vi "CaculateDivergenceAngle .vi"(3 "位置路径":path[](array[path])) -> (0 "纵向发散角":dbl, 1 "横向发散角":dbl)   [LabVIEW 2018]
panel:
  out "Image":T1(plugin-control)
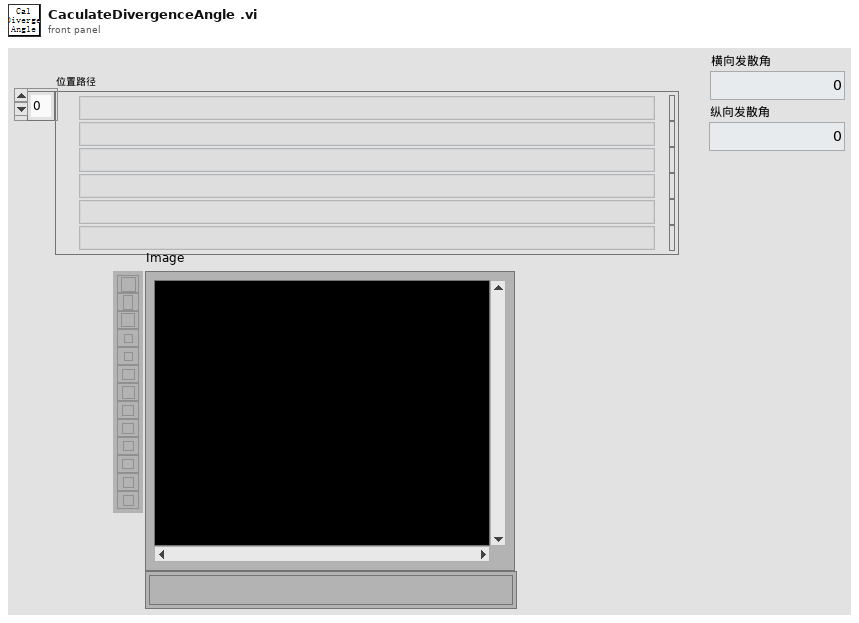
[diagram p1: front panel]
types:
  T1 = typedef "IMAQ Image.ctl" = refnum<image>
  T2 = cluster{"示波器":cluster{"Channel (0:Channel 1)":enum16{"Channel 1", "Channel 2", "Channel 3", "Channel 4"}, "电压范围":dbl, "触发电压":dbl, "时间范围":dbl, " 示波器VISA":refnum<visa-resource-name>, "时间范围 标签":u64, "电压范围 标签":u64, "触发电压 标签":u64}, "光谱仪":cluster{"SpecDataReference":refnum<queue>, "grating center":dbl, "Exposure Time (s)":dbl, "是否进行详细设置":bool, " 开始通信检查":bool, "通信成功？":bool, "波长":dbl}, " 近场相机":cluster{"曝光时间/100us":dbl, "模拟增益":i32, "控制套接字":i32, "IP 地址":string, " 采集套接字":i32, "  版本号":i32, "ImageData":T1, "  增益最大":i32, "  增益最小":i32, " 曝光最大":i32, " 曝光最小":i32, " 帧速":i32, " 同步切换":i32, "  曝光缩放":i32}, " 偏振仪":cluster{"电压范围":u64, "触发电压":u64, "时间范围":u64, "波长范围":enum16{"可见光 400-700nm", "近红外 700-1100nm"}, "可见光偏振测量仪VISA":refnum<visa-resource-name>, "近红外偏振测量仪VISA":refnum<visa-resource-name>}, " 功率计":cluster{"通道":enum16{"Channel 1", "Channel 2"}, "工作波长":u32, "单位":u64, "时间范围":u64, "IP地址":string, "端口":u32}, "能量计":cluster{"通道":enum16{"Channel 1", "Channel 2"}, "工作波长":u32, "单位":u64, "时间范围":u64, "IP地址":string, "端口":u32, "能量计量程":enum16{"200uJ", "20uJ", "2uJ", "200nJ"}}, "电机":cluster{"Channel (0:Channel 1)":enum16{"Channel 1", "Channel 2", "Channel 3", "Channel 4"}, "电压范围":u64, "触发电压":u64, "时间范围":u64}, " 远场相机":cluster{"曝光时间":i32, "模拟增益":i32, "控制套接字":i32, "IP 地址":string, " 采集套接字":i32, "  版本号":i32, "ImageData":T1, "  增益最大":i32, "  增益最小":i32, " 曝光最大":i32, " 曝光最小":i32, " 帧速":i32, " 同步切换":i32, "  曝光缩放":i32, "ImageData B":T1}}
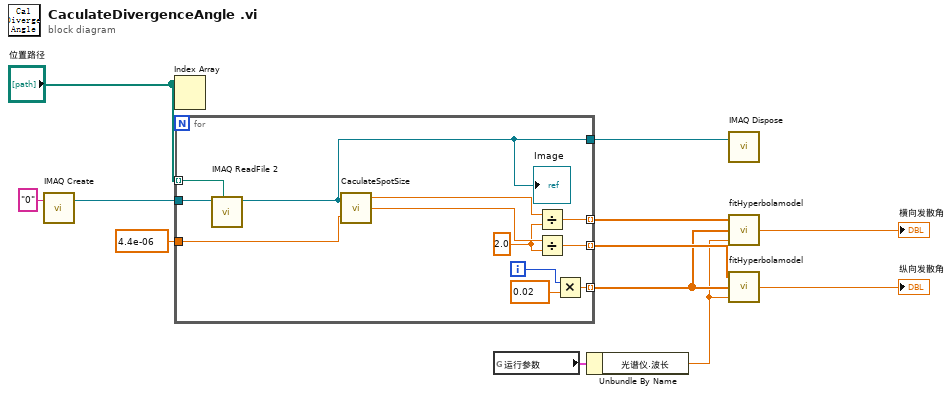
[diagram p0: block diagram]
diagram:
  n1 = call "IMAQ Create"("Image Name"="0") -> ("New Image"=w10:T1)  [unwired: 4 in, 1 out]
  n2 = Index Array(array="位置路径") -> ()  [unwired: 2 in, 2 out]
  n3 = for {
    tunnel: "位置路径" -> [w14] mode=indexing
    tunnel: w10 -> [w24]
    tunnel: 4.4e-06 ("单个像元大小") -> [w23]
    tunnel: [w20] -> w4 mode=indexing
    tunnel: [w18] -> w7 mode=indexing
    tunnel: [w15] -> w5 mode=indexing
    tunnel: [w13] -> w8
    i -> [w22]
    w16 = 2.0 ("y")
    n4 = call "IMAQ ReadFile 2"("File Path"=w14, "Image"=w24) -> ("Image Out"=w13:T1)  [unwired: 5 in, 4 out]
    "Image" <- w13
    n5 = call "CaculateSpotSize .vi"("图像输入"=w13, "单个像元大小"=w23) -> ("光斑横向大小"=w19:dbl, "光斑纵向大小"=w17:dbl)  [unwired: 1 out]
    n6 = Divide(x=w19, y=w16) -> (x/y=w18:dbl)
    n7 = Divide(x=w17, y=w16) -> (x/y=w15:dbl)
    n8 = Multiply(x=w22, y=0.02) -> (x*y=w20:dbl)
  }
  n9 = global read "参数.vi" "运行参数"() -> (w3:T2)
  n10 = Unbundle By Name(w3) -> ("光谱仪.波长"=w2:dbl)
  n11 = call "IMAQ Dispose"("Image"=w8) -> ()  [unwired: 5 in, 1 out]
  n12 = call "fitHyperbolamodel.vi"("lambda"=w2, "Z"=w4, "Wz"=w7) -> ("发散角"=→"横向发散角":dbl)  [unwired: 2 in]
  n13 = call "fitHyperbolamodel.vi"("lambda"=w2, "Z"=w4, "Wz"=w5) -> ("发散角"=→"纵向发散角":dbl)  [unwired: 2 in]
